vi "PAN_RunCmdSet.vi"(8 "error in (no error)":errorcluster, 10 "cmd in":string, 11 "type specifier VI Refnum (for type only)":refnum<vi>) -> (0 "error out":errorcluster, 2 "cmd out":string, 3 "type specifier out":refnum<vi>)   [LabVIEW 2016]
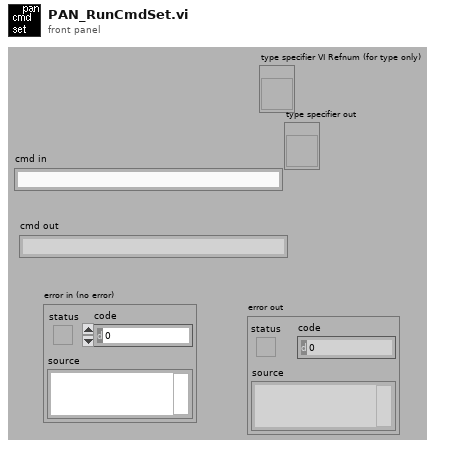
[diagram p1: front panel]
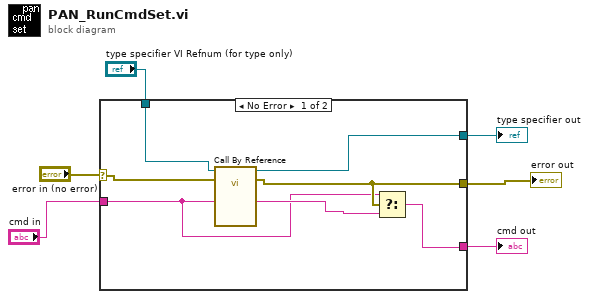
[diagram p0: block diagram]
diagram:
  n1 = case shown="No Error" "error in (no error)" {
    selector: "error in (no error)" -> [w13 w16]
    tunnel: [w10 w16] -> w6
    tunnel: "cmd in" -> [w8 w15]
    tunnel: [w7 w15] -> w4
    tunnel: "type specifier VI Refnum (for type only)" -> [w12 w14]
    tunnel: [w11 w14] -> w1
    frame No Error {
      n2 = call-by-ref "?"(reference=w12, error in=w13, "cmd in"=w8) -> (reference out=w11:refnum<vi>, error out=w10:errorcluster, "cmd out"=w9:string)  [unwired: 10 in]
      n3 = Select(t=w8, s=w10, f=w9) -> (s? t:f=w7:string)
    }
    frame Error {
    }
  }
  "error out" <- w6
  "cmd out" <- w4
  "type specifier out" <- w1
